vi "Read Lockin Digitizer Configuration.vi"(8 "error in (no error)":errorcluster, 11 "DAQmx Lockin Digitizer Driver in":refnum<class "Lockin Digitizer Driver.lvclass">) -> (0 "error out":errorcluster, 2 "Configuration":T1={"Post-trigger delay"=0.01, "Post-trigger duration"=0.1, "Rate"=1000000.0, "Ranges"=[10.0], "Re-name channels"=[], "Active channels"="0:1", "External\nclock"=FALSE, "Monitor time\nconstant"=1.0, "Sync"=FALSE, "Lock-in input channel phases"=[], "Output channels configuration"=[]} {"Output channels configuration"."Output amplitude" format="%#_6pV"; "Output channels configuration"."Frequency" format="%#_6pHz"; "Monitor time\nconstant" format="%#_6ps"; "Rate" format="%#_8pHz"; "Post-trigger duration" format="%#_6ps"; "Post-trigger delay" format="%#_6ps"; "Ranges" format="%#_6pV"}, 3 "DAQmx Lockin Digitizer Driver in":refnum<class "Lockin Digitizer Driver.lvclass">)   [LabVIEW 2024, in "Lockin Digitizer Driver.lvclass"]
uses:
  Lockin Digitizer Driver.lvclass
  Lockin Digitizer Configuration.ctl
  Lockin Digitizer Driver.lvclass/Lockin Digitizer Driver.ctl
  Lockin Digitizer Driver/Output Channel Configuration.ctl
panel:
  # "Pulse config"
  # "Lock-in config"
  # "Output        Output          Input\nfrequency    amplitude    channels"
  # "#0\n\n#1\n\n#3"
  # "Monitor config"
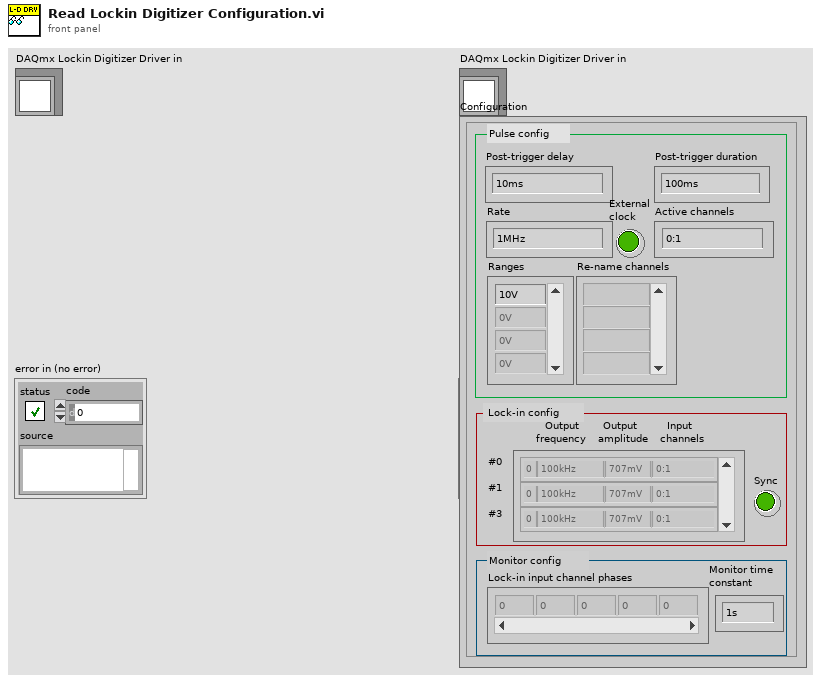
[diagram p1: front panel]
types:
  T1 = typedef "Lockin Digitizer Configuration.ctl" = cluster{"Post-trigger delay":dbl, "Post-trigger duration":dbl, "Rate":dbl, "Ranges":dbl[], "Re-name channels":string[], "Active channels":string, "External\nclock":bool, "Monitor time\nconstant":dbl, "Sync":bool, "Lock-in input channel phases":dbl[], "Output channels configuration":T2[]}
  T2 = typedef "Output Channel Configuration.ctl" = cluster{"Input channels":string, "Frequency":dbl, "Output amplitude":dbl, "Output channel number":i32}
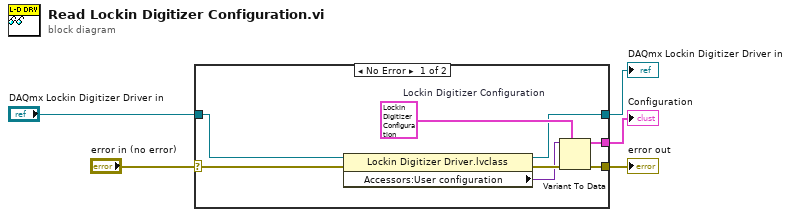
[diagram p0: block diagram]
diagram:
  n1 = case shown="No Error" "error in (no error)" {
    selector: "error in (no error)" -> [w12 w14]
    tunnel: [w11 w14] -> w4
    tunnel: [w7 w15] -> w2
    tunnel: "DAQmx Lockin Digitizer Driver in" -> [w8 w15]
    tunnel: [w10 _] -> w1
    frame No Error {
      w13 = T1 {"Post-trigger delay"=0.01, "Post-trigger duration"=0.1, "Rate"=1000000.0, "Ranges"=[10.0], "Re-name channels"=[], "Active channels"="0:1", "External\nclock"=FALSE, "Monitor time\nconstant"=1.0, "Sync"=FALSE, "Lock-in input channel phases"=[], "Output channels configuration"=[]}  # Lockin Digitizer Configuration
      n2 = property class="Lockin Digitizer Driver.lvclass"(reference=w8, error in=w12) -> (reference out=w7:refnum<class "Lockin Digitizer Driver.lvclass">, error out=w9:errorcluster, "Accessors:User configuration"=w6:variant)
      n3 = Variant To Data(error in=w9, type=w13, Variant=w6) -> (data=w10:T1, error out=w11:errorcluster)
    }
    frame Error {
    }
  }
  "error out" <- w4
  "DAQmx Lockin Digitizer Driver in" <- w2
  "Configuration" <- w1
